vi "SoS_Kc_2024.vi"(3 "xw H2O molar fraction":dbl, 4 "Temperature [K]":dbl=293.15 format="%#.4g", 5 "CO2 content (ppm)":dbl=500.0, 6 "Type of air":i32(listbox)=4) -> (0 "Kc":dbl=-0.0010172235386579631, 1 "Sos gamma0RT/M check [m/s]":dbl=343.2297660564569 format="%.4g", 2 "Sos Kc (m/s)":dbl=343.22976605645687 format="%.4f")   [LabVIEW 2016]
panel:
  out "Kc (ppm)":dbl=-1017.2235386579631
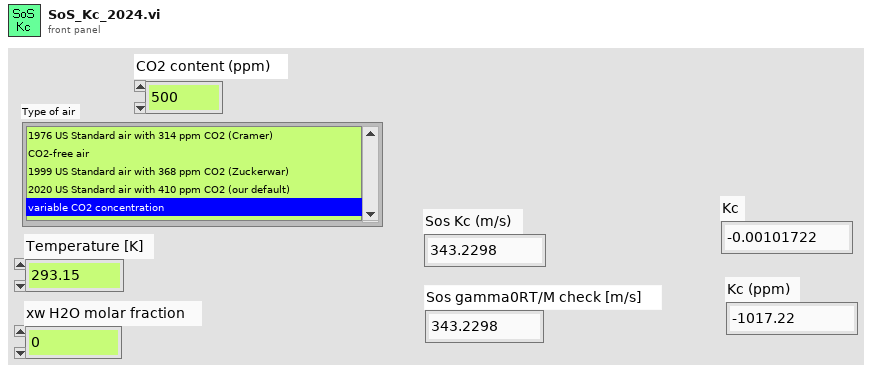
[diagram p1: front panel]
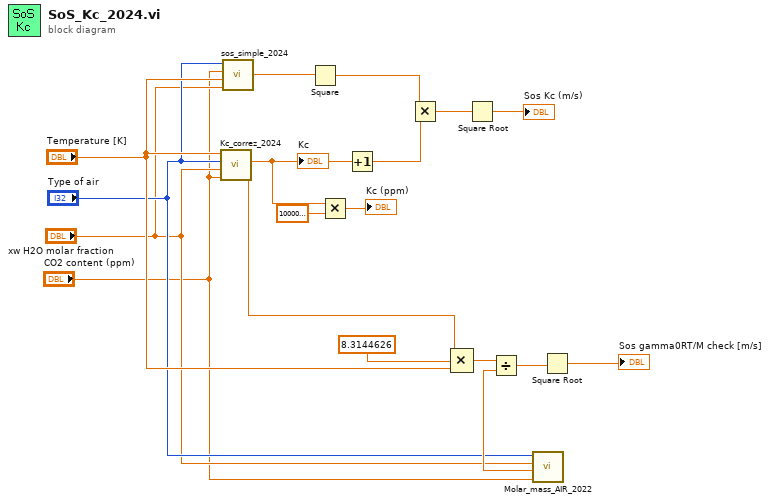
[diagram p0: block diagram]
diagram:
  n1 = call "Kc_correz_2024.vi"("Temperature [K]"="Temperature [K]", "Type of air"="Type of air", "H2O molar fraction"="xw H2O molar fraction", "CO2 content (ppm)"="CO2 content (ppm)") -> ("Kc - correction"=w3:dbl, "Gamma0 humid air"=w10:dbl)  [unwired: 4 out]
  "Kc" <- w3
  n2 = call "sos_simple_2024.vi"("xw H2O molar fraction"="xw H2O molar fraction", "Temperature [K]"="Temperature [K]", "CO2 content (ppm)"="CO2 content (ppm)", "Type of air"="Type of air") -> ("Simple speed of sound  correct [m/s]"=w9:dbl)  [unwired: 1 out]
  n3 = Square(x=w9) -> (x^2=w8:dbl)
  n4 = Multiply(x=w3, y=1000000.0) -> (x*y=→"Kc (ppm)":dbl)
  n5 = Increment(x=w3) -> (x+1=w18:dbl)
  n6 = Multiply(x=w8, y=w18) -> (x*y=w17:dbl)
  n7 = Compound Arithmetic op=MULTIPLY(w10, 8.3144626, "Temperature [K]") -> (w16:dbl)
  n8 = Square Root(x=w17) -> (sqrt(x)=→"Sos Kc (m/s)":dbl)
  n9 = call "Molar_mass_AIR_2022.vi"("CO2 content (ppm)"="CO2 content (ppm)", "xw molar fraction of water vapor"="xw H2O molar fraction", "Type of air"="Type of air") -> ("Molar mass humid air [kg/mol]"=w12:dbl)  [unwired: 8 out]
  n10 = Divide(x=w16, y=w12) -> (x/y=w15:dbl)
  n11 = Square Root(x=w15) -> (sqrt(x)=→"Sos gamma0RT/M check [m/s]":dbl)
